vi "csafePIP.vi"(8 "error in (no error)":errorcluster) -> (0 "error out":errorcluster, 3 "CSAFE-21":string)   [LabVIEW 2018]
uses:
  Global_1259.vi
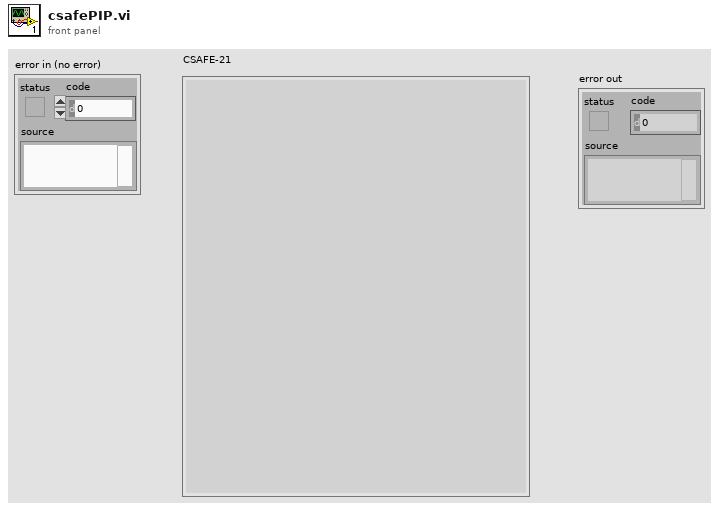
[diagram p1: front panel]
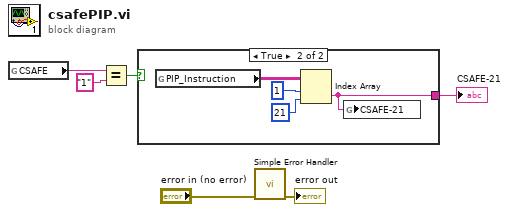
[diagram p0: block diagram]
diagram:
  n1 = global read "Global_1259.vi" "CSAFE"() -> (w3:string)
  n2 = Equal?(x=w3, y="1") -> (x = y?=w5:bool)
  n3 = case shown="True" w5 {
    tunnel: [_ w7] -> w6
    frame False {
    }
    frame True {
      n4 = global read "Global_1259.vi" "PIP_Instruction"() -> (w10:string[][])
      n5 = Index Array(array=w10, index (row)=1, index (col)=21 ("disabled index (col)")) -> (element=w7:string)
      n6 = global write "Global_1259.vi" "CSAFE-21"(w7) -> ()
    }
  }
  "CSAFE-21" <- w6
  n7 = call <vilib>:"Simple Error Handler.vi"("error in (no error)"="error in (no error)") -> ("error out"=→"error out":errorcluster)  [unwired: 4 in, 4 out]
